vi "is_code_plus_eco.vi"(4 "code":i32) -> (1 "has + ECO?":bool)   [LabVIEW 2015]
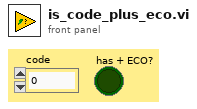
[diagram p1: front panel]
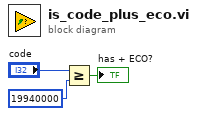
[diagram p0: block diagram]
diagram:
  n1 = Greater Or Equal?(x="code", y=19940000 ("lower limit")) -> (x >= y?=→"has + ECO?":bool)
